vi "Send Error to Notebook.vi"(8 "error in (no error)":errorcluster, 9 "Verbose Error Messages (T)":bool=TRUE, 10 "State Machine Case Error Source":string, 11 "Notebook Q":refnum<queue>) -> (0 "Error Out":errorcluster)   [LabVIEW 2021, in "Notebook.lvlib"]
uses:
  Notebook.lvlib
  Notebook Action Q Element.ctl
  Notebook Action List.ctl
  Notebook Parameters List.ctl
  <userlib>/_OpenG.lib/error/error.llb/Filter Error Codes (Array)__ogtk.vi
  Variant/Variant to Data/Variant to Boolean.vi
  Rich Text Box/Rich Text Box.lvlib
  Strings/Strings.lvlib
  Variant/Variant to Data/Variant to Data.lvlib
  <userlib>/_OpenG.lib/error/error.llb/openg_error.lvlib
  Sound/Sound.lvlib
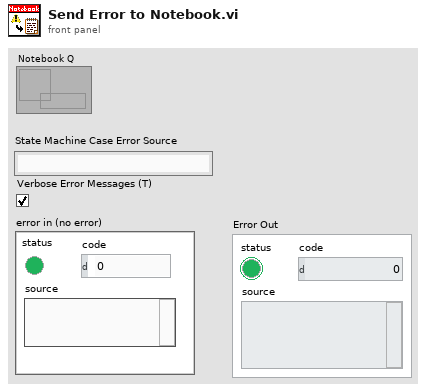
[diagram p1: front panel]
types:
  T1 = typedef "Notebook.lvlib/Notebook Parameters List.ctl" = enum16{"First Opening?", "Saved Notebook?", "Saved Notebook Path", "Beep on Error?"}
  T2 = typedef "Rich Text Box.lvlib/Text Formatting.ctl" = cluster{"Font":string, "Text Color":T3, "Text Background Color":T3, "Text Style":enum16{"Regular", "Bold", "Italic", "Underline", "Strikeout"}, "Font Size (Points)":dbl, "Text Alignment":i32}
  T3 = typedef "Rich Text Box.lvlib/Text Colors.ctl" = enum16{"Unchanged", "Black", "Blue", "Brown", "Gray", "Green", "Orange", "Pink", "Red", "White"}
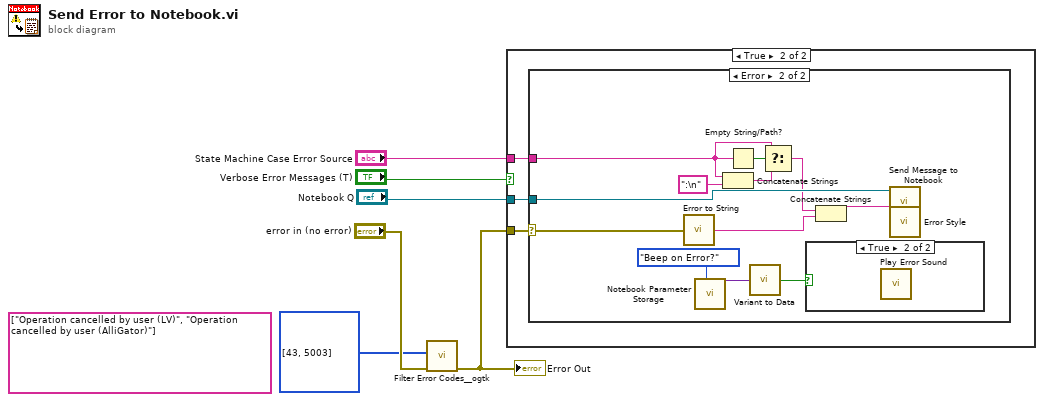
[diagram p0: block diagram]
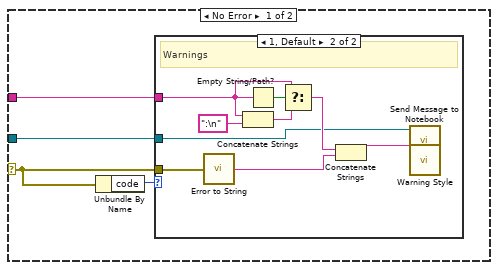
[diagram p3: hidden frame]
diagram:
  (unwired) string[] ["Operation cancelled by user (LV)", "Operation cancelled by user (AlliGator)"]
  n1 = call-poly <userlib>:"Filter Error Codes__ogtk.vi"("Error In"="error in (no error)", "Error Codes to Filter"=i32[] [43, 5003]) -> ("Error Out"=w2:errorcluster)  [unwired: 7 in, 2 out]
  "Error Out" <- w2
  n2 = case shown="True" "Verbose Error Messages (T)" {
    tunnel: "Notebook Q" -> [_ w9]
    tunnel: "State Machine Case Error Source" -> [_ w8]
    tunnel: w2 -> [_ w7]
    frame False {
    }
    frame True {
      n3 = case shown="Error" w7 {
        selector: w7 -> [w11 w34]
        tunnel: w9 -> [w13 w36]
        tunnel: w8 -> [w10 w35]
        frame No Error {
          n4 = Unbundle By Name(w11) -> ("code"=w12:i32)
          n5 = case shown="1, Default" w12 {
            tunnel: w13 -> [_ w17]
            tunnel: w11 -> [_ w16]
            tunnel: w10 -> [_ w15]
            frame 0 {
            }
            frame 1, Default {
              # "Warnings"
              n6 = call "Error to String.vi"("error in (no error)"=w16) -> ("message"=w18:string)  [unwired: 8 in]
              n7 = Concatenate Strings(w15, ":\n" ("string")) -> (w19:string)
              n8 = Empty String/Path?(string/path=w15) -> (empty?=w22:bool)
              n9 = Select(t=w15, s=w22, f=w19) -> (s? t:f=w21:string)
              n10 = Concatenate Strings(w21, w18) -> (w23:string)
              n11 = call "Warning Style.vi"() -> ("Error Formatting"=w14:T2)
              n12 = call "Send Message to Notebook.vi"("Text Formatting"=w14, "Message"=w23, "Notebook Queue"=w17) -> ()  [unwired: 5 in, 2 out]
            }
          }
        }
        frame Error {
          n13 = call "Error to String.vi"("error in (no error)"=w34) -> ("message"=w28:string)  [unwired: 8 in]
          n14 = call "Notebook Parameter Storage.vi"("Notebook Parameter List"=Notebook_Parameters_List."Beep on Error?") -> ("Data out"=w25:variant)  [unwired: 9 in, 1 out]
          n15 = Concatenate Strings(w35, ":\n" ("string")) -> (w29:string)
          n16 = Empty String/Path?(string/path=w35) -> (empty?=w32:bool)
          n17 = call-poly "Variant to Data.vi"("Variant"=w25) -> ("Value"=w26:bool)  [unwired: 8 in]
          n18 = Select(t=w35, s=w32, f=w29) -> (s? t:f=w31:string)
          n19 = case shown="True" w26 {
            frame False {
            }
            frame True {
              n20 = call "Play Error Sound.vi"() -> ()  [unwired: 27 in, 1 out]
            }
          }
          n21 = Concatenate Strings(w31, w28) -> (w33:string)
          n22 = call "Error Style.vi"() -> ("Error Formatting"=w27:T2)
          n23 = call "Send Message to Notebook.vi"("Text Formatting"=w27, "Message"=w33, "Notebook Queue"=w36) -> ()  [unwired: 5 in, 2 out]
        }
      }
    }
  }
